vi "Max Current.vi"() -> (0 "y":dbl=500.0 format="%#_13g")   [LabVIEW 2015]
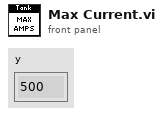
[diagram p1: front panel]
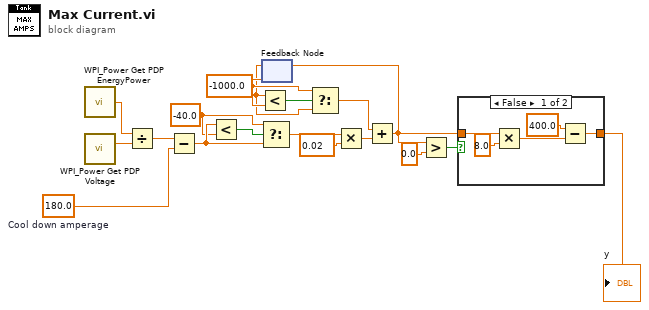
[diagram p0: block diagram]
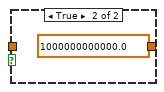
[diagram p2: hidden frame]
diagram:
  w12 = -40.0 ("y")
  w15 = 180.0  # Cool down amperage
  w10 = -1000.0
  n1 = call <vilib>:"WPI_Power Get PDP EnergyPower.vi"() -> ("Power (W)"=w18:dbl)  [unwired: 13 in, 2 out]
  n2 = call <vilib>:"WPI_Power Get PDP Voltage.vi"() -> ("voltage (V)"=w17:dbl)  [unwired: 14 in, 1 out]
  n3 = Divide(x=w18, y=w17) -> (x/y=w16:dbl)
  n4 = Subtract(x=w16, y=w15) -> (x-y=w13:dbl)
  n5 = Less?(x=w13, y=w12) -> (x < y?=w14:bool)
  n6 = Select(t=w12, s=w14, f=w13) -> (s? t:f=w6:dbl)
  n7 = feedback #1(w10) -> (w9:dbl)
  n8 = Less?(x=w9, y=w10) -> (x < y?=w11:bool)
  n9 = Select(t=w10, s=w11, f=w9) -> (s? t:f=w8:dbl)
  n10 = Multiply(x=w6, y=0.02) -> (x*y=w5:dbl)
  n11 = Add(x=w8, y=w5) -> (x+y=w2:dbl)
  n12 = feedback-in #1(w2) -> ()
  n13 = Greater?(x=w2, y=0.0) -> (0:w3:bool)
  n14 = case shown="False" w3 {
    tunnel: w2 -> [w21 _]
    tunnel: [w19 1000000000000.0] -> w1
    frame False {
      n15 = Multiply(x=w21, y=8.0) -> (x*y=w20:dbl)
      n16 = Subtract(x=400.0, y=w20) -> (x-y=w19:dbl)
    }
    frame True {
    }
  }
  "y" <- w1
